vi "Measurement UI.vi"() -> ()   [LabVIEW 2022 SP3, in "Single Tone - Digital Mic UI.lvlib"]
uses:
  Single Tone - Digital Mic UI.lvlib
  shared/measurements/controls/measurement units.ctl
  shared/ui/controls/view.ctl
  shared/controls/input type.ctl
  UI State.ctl
  <vilib>/Utility/miscctls.llb/LVBoundsTypeDef.ctl
  <vilib>/Utility/miscctls.llb/LVPoint32TypeDef.ctl
  <vilib>/Utility/miscctls.llb/LVPointTypeDef.ctl
  shared/ui/UI Helpers.lvlib
  shared/configuration dialogs/Config Dialog.lvlib
panel:
  in  "view legend":T1
  out "time domain":waveform(dbl)[](graph)
  out "frequency domain":cluster{"x0":dbl, "dx":dbl, "magnitude":dbl[]}[](graph)
  out "meas table":string[][](table)
  out "THD":dbl caption="frequency (Hz) 3"
  out "THD+N":dbl caption="frequency (Hz) 2"
  out "SNR":dbl
  out "microphone sensitivity (dBFS)":dbl
  out "amplitude (dBSPL)":dbl
  out "amplitude (Pa RMS)":dbl
  out "frequency (Hz)":dbl
  out "channel name":string
  out "ref mic wfm - data":dbl[](array[numeric])
  out "ref mic wfm - dt":dbl
  in  "output channel":string="PXI1Slot4/ai0"
  in  "input cfg file":string
  in  "Configuration tab":enum32{"Input", "Measurement", "Units"}(tab)=enum."Measurement"
  in  "digital mic sensitivity (dBFS)":dbl=-26.0 caption="Microphone Sensitivity" format="%#.6p dBFS"
  out "input cfg file name":string
  in  "configure input":bool
  in  "digital channel list":string="PXI1Slot2\\PCMi 0" caption="Digital Audio Channel"
  in  "input type":T2 caption="Input Type"
  in  "Output Channel":tag="PXI1Slot2/ao0" caption="Channel"
  in  "output level (dBSPL)":dbl=94.0 caption="Output level" format="%#_3f dBSPL"
  in  "min settling cycles":u32 caption="Minimum settling cycles"
  in  "min settling time (s)":dbl=0.1 caption="Minimum settling time" format="%#_6ps"
  in  "min measurement cycles":u32 caption="Minimum measurement cycles"
  in  "min measurement time (s)":dbl=0.1 caption="Minimum measurement time" format="%#_6ps"
  in  "Ref Mic Channel":tag="PXI1Slot2/ai0" caption="Channel"
  in  "acq sampling rate":dbl=50.0 caption="Sensitivity" format="%#.6f mV/Pa"
  in  "lowpass filter":T3(ring) caption="Lowpass filter"
  in  "highpass filter":enum32{"DC", "AC"}(ring)=enum."AC" caption="Highpass filter"
  in  "band start":dbl=20.0 caption="Band start" format="%#_6pHz"
  in  "band stop":dbl=20000.0 caption="Band stop" format="%#_6pHz"
  in  "weighting filter":T4(ring)=enum."A-weighting" caption="Weighting filter"
  in  "output voltage ratio":dbl=3.39 caption="Output voltage ratio" format="%.3p Pa/V"
  in  "signal frequency":dbl=1000.0 caption="Frequency" format="%#_6pHz"
  in  "THD units":T5 caption="THD"
  in  "THD+N units":T5 caption="THD+N"
  in  "SNR units":T5 caption="SNR"
  out "fft - data":dbl[](array[numeric])
  out "fft - df":dbl
  out "fft - f0":dbl
  out "wfm - data":dbl[](array[numeric])
  out "wfm - dt":dbl
  in  "ref mic channel":string="PXI1Slot4/ai0"
  # "hidden controls - used to sync with MeasLink"
  # "hidden indicators"
  # "Digital Microphone Interface"
  # "Harware Resource"
  # "Output"
  # "Reference Microphone"
  # "Measurement Duration"
  # "Filters"
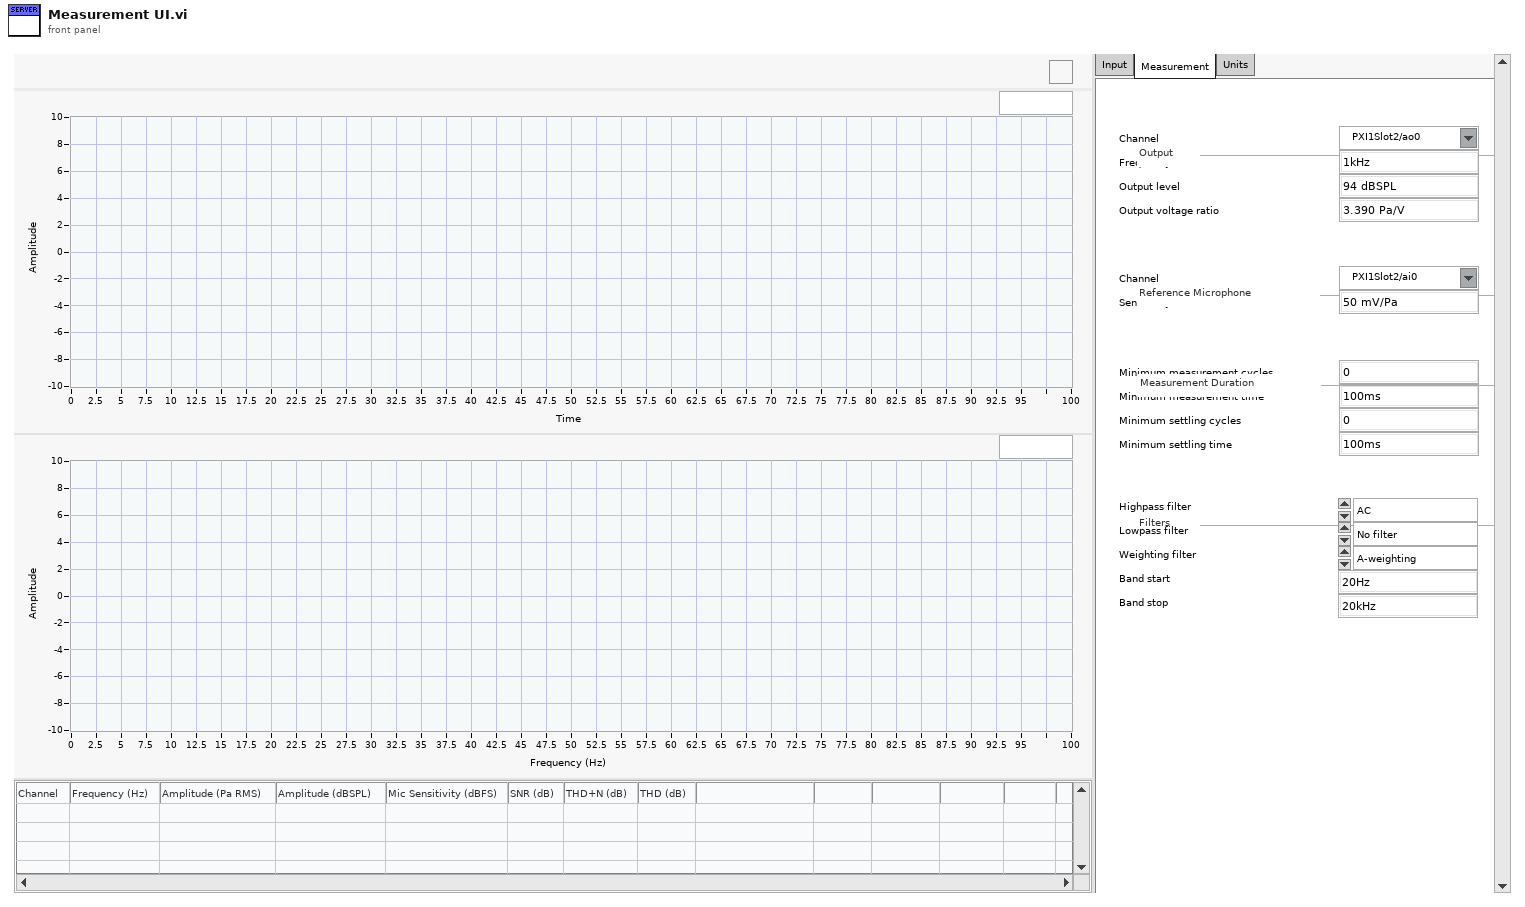
[diagram p1: front panel]
types:
  T1 = typedef "UI Helpers.lvlib/view.ctl" = bool
  T2 = typedef "input type.ctl" = enum32{"Digital Serial", "PDM"}
  T3 = enum32{"No filter", "AES17 20kHz", "AES17 40kHz"}
  T4 = enum32{"Linear", "A-weighting", "B-weighting", "C-weighting"}
  T5 = typedef "measurement units.ctl" = enum32{"dB", "%", "x/y"}
  T6 = typedef "Single Tone - Digital Mic UI.lvlib/UI State.ctl" = cluster{"Graph Size":T7, "Legend Visible":bool, "Mouse Coords":T8, "PostUI event occurred":bool, "input cfg file":path}
  T7 = typedef "LVBoundsTypeDef.ctl" = cluster{"Width":u32, "Height":u32}
  T8 = typedef "LVPoint32TypeDef.ctl" = cluster{"Horizontal":i32, "Vertical":i32}
  T9 = typedef "LVPointTypeDef.ctl" = cluster{"Horizontal":i16, "Vertical":i16}
  T10 = typedef "Config Dialog.lvlib/audio settings.ctl" = cluster{"input cfg file":string}
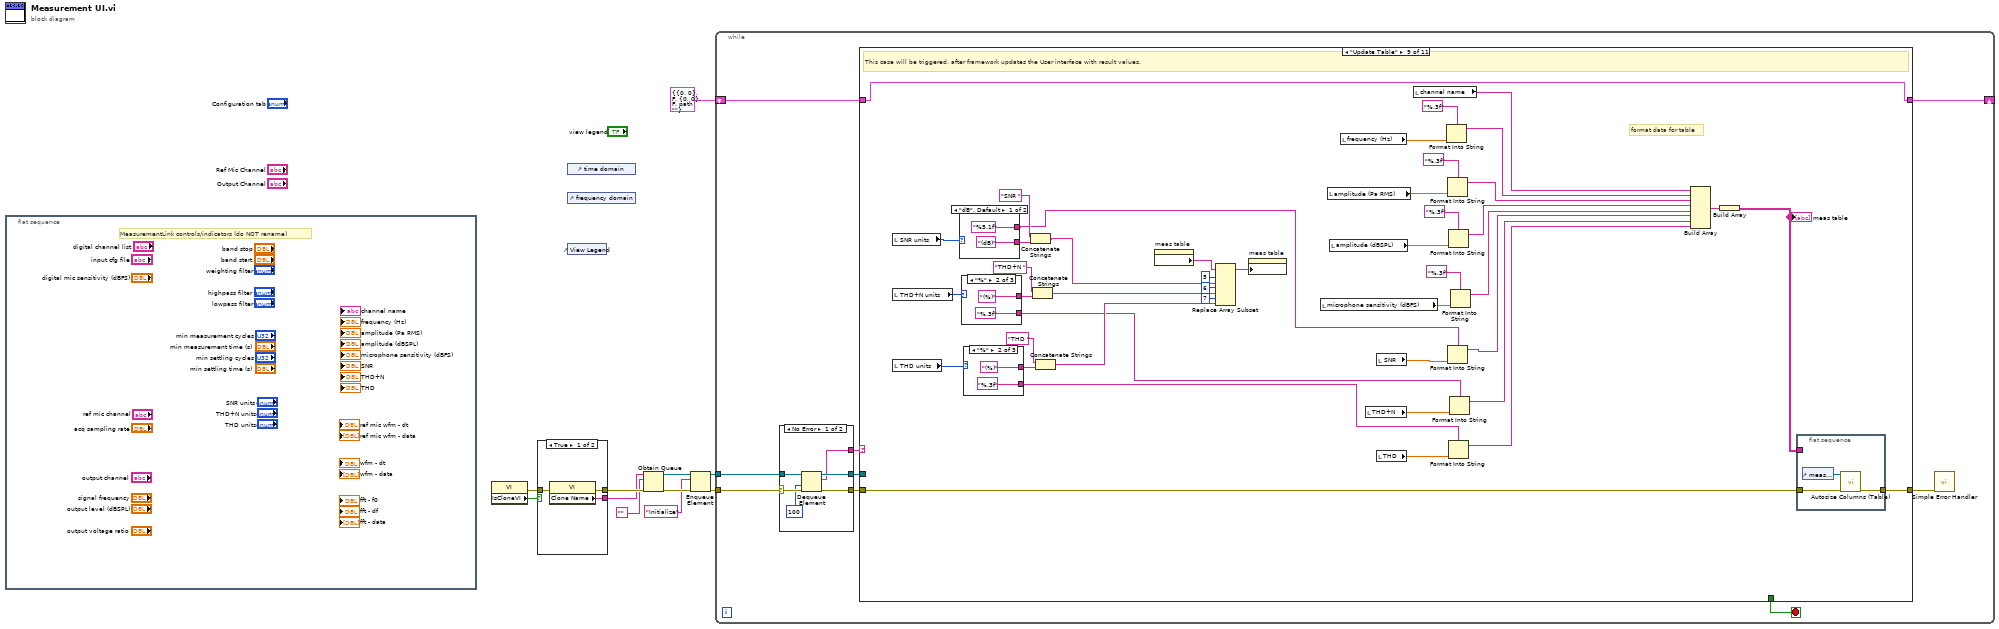
[diagram p0: block diagram]
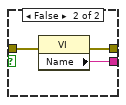
[diagram p2: hidden frame]
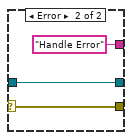
[diagram p3: hidden frame]
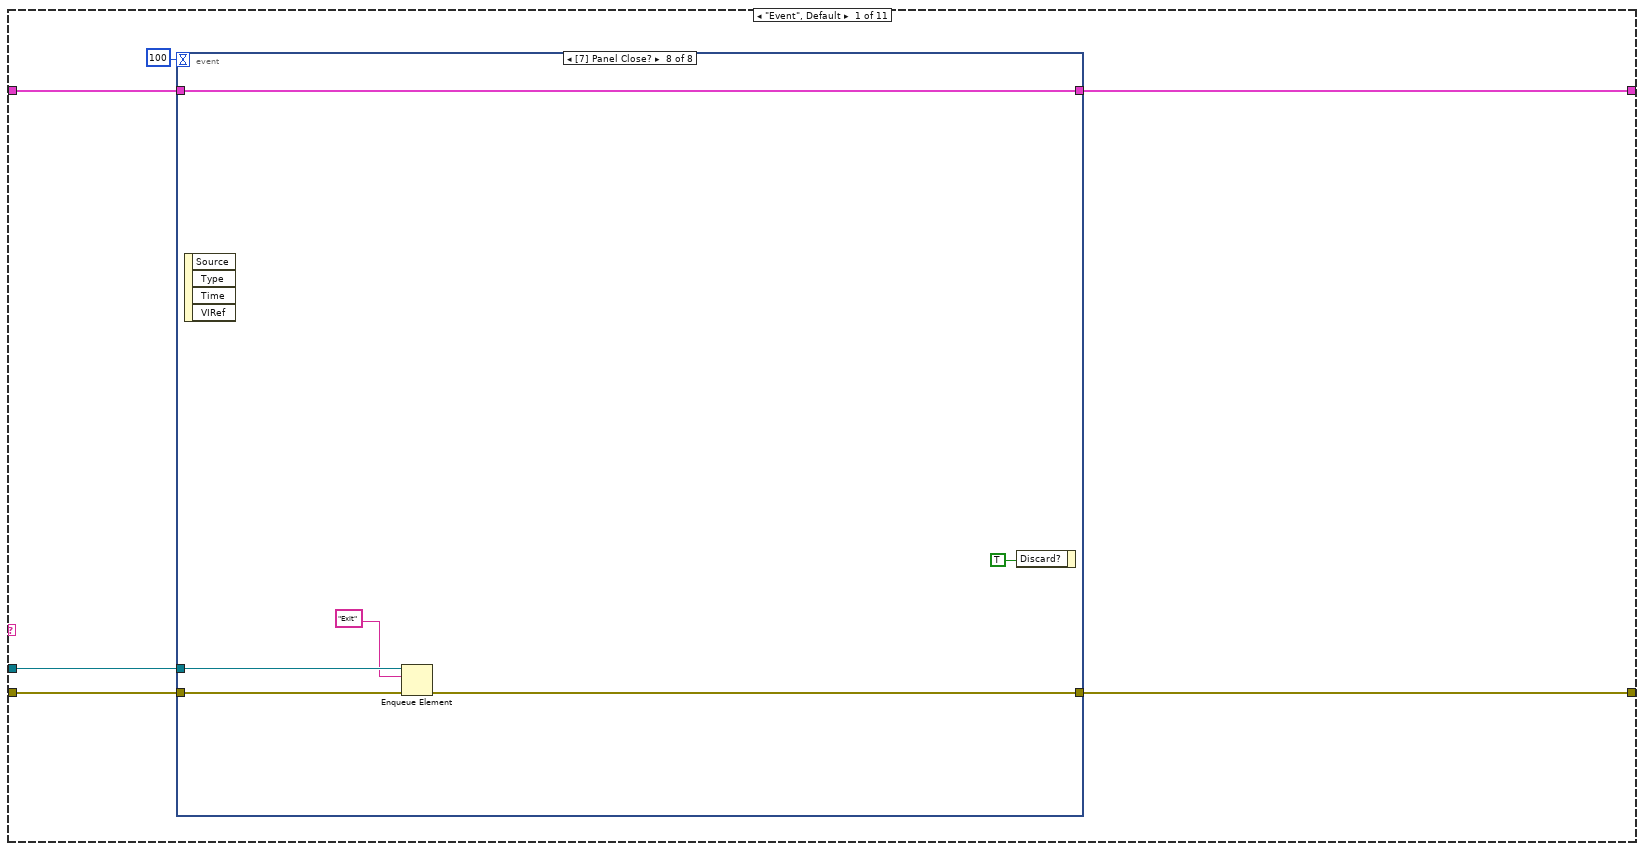
[diagram p4: hidden frame]
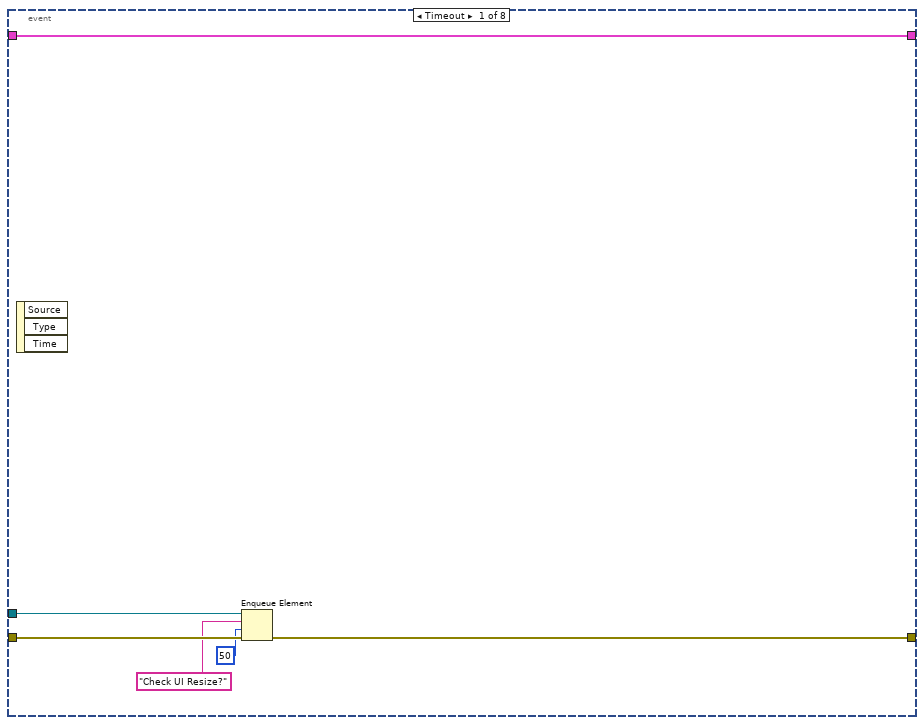
[diagram p5: hidden frame]
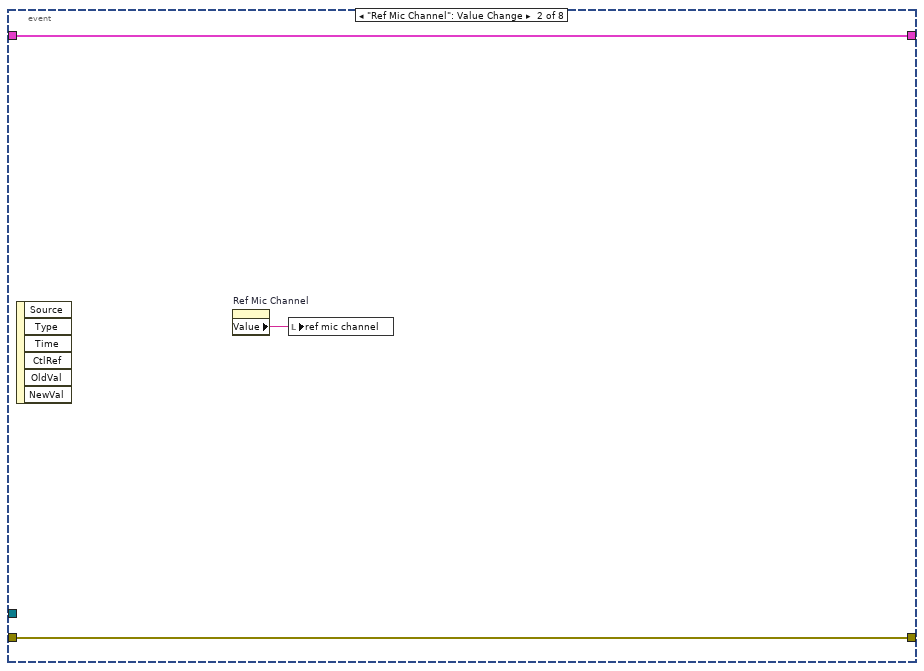
[diagram p6: hidden frame]
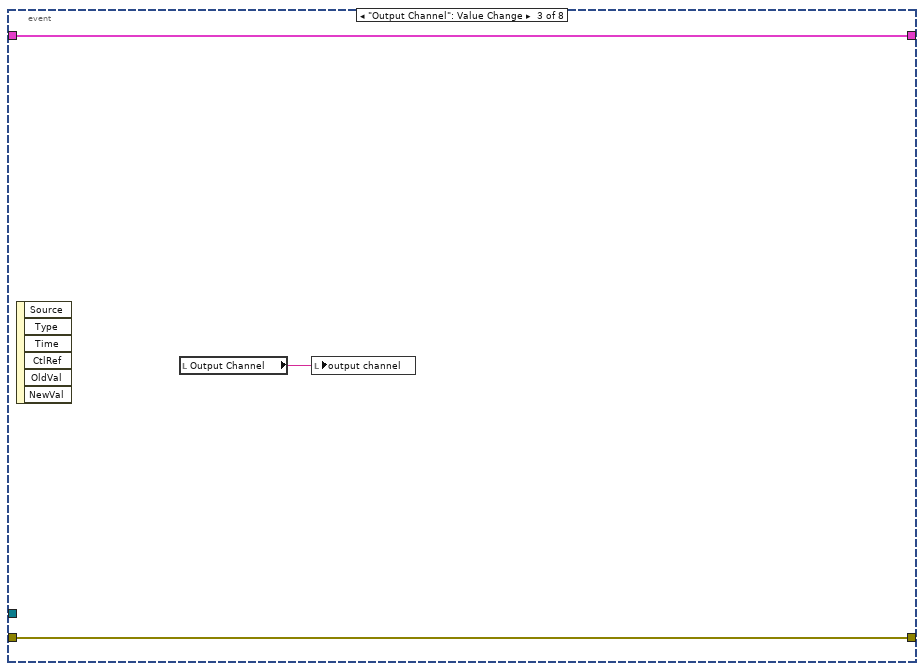
[diagram p7: hidden frame]
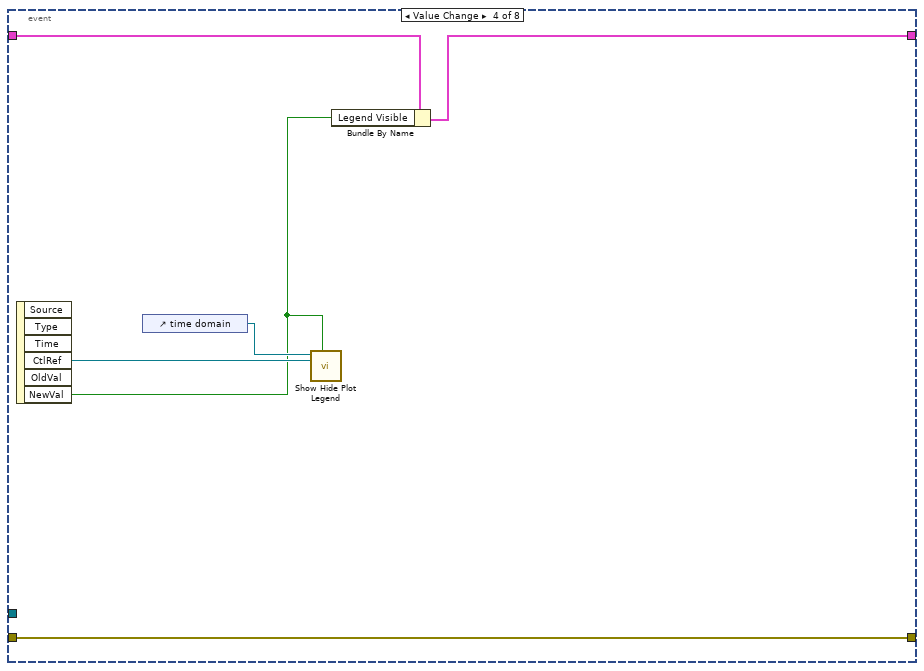
[diagram p8: hidden frame]
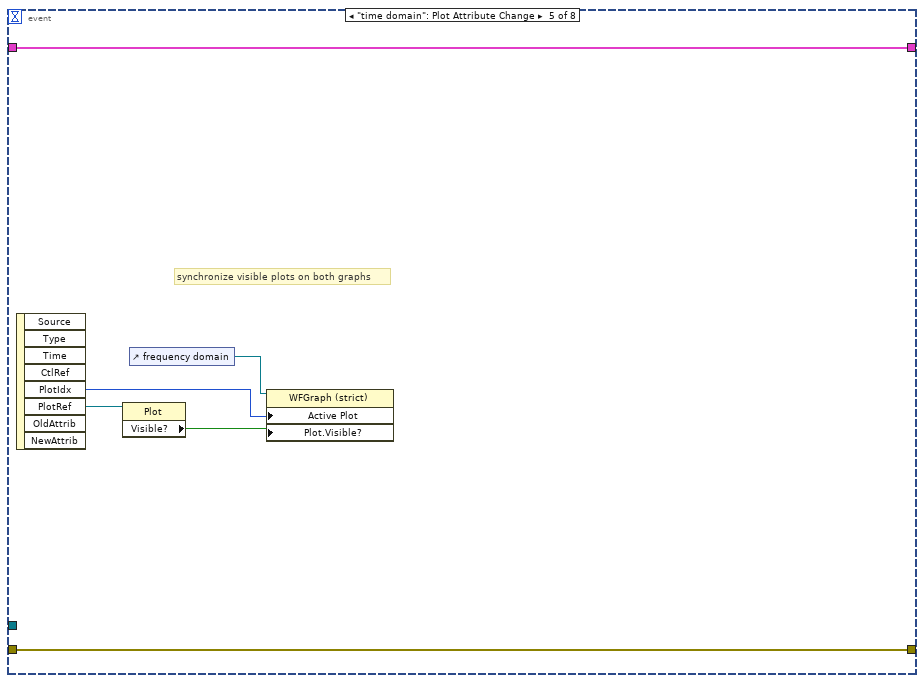
[diagram p9: hidden frame]
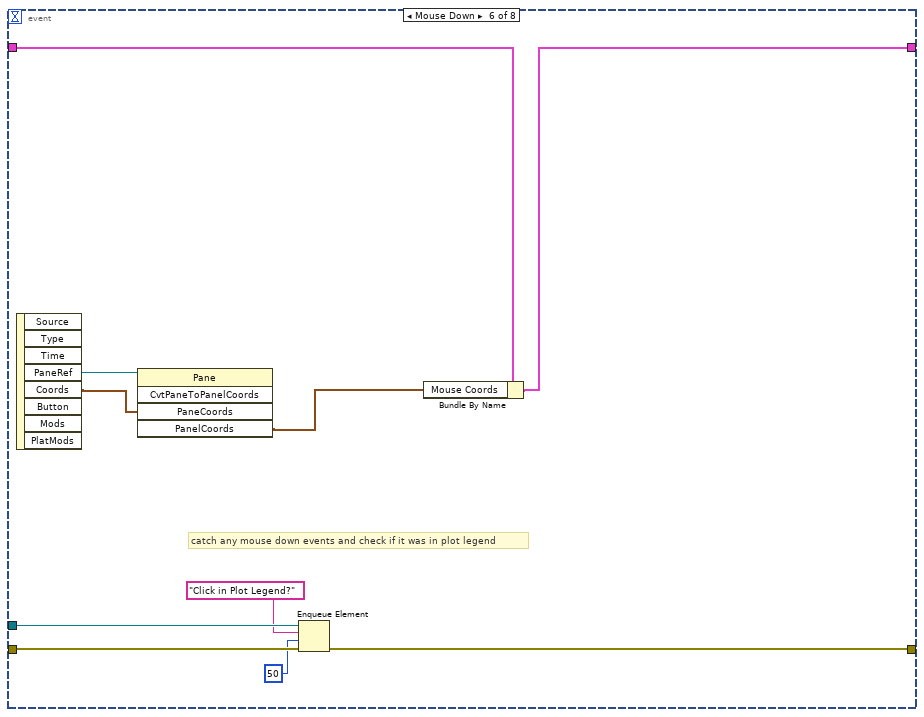
[diagram p10: hidden frame]
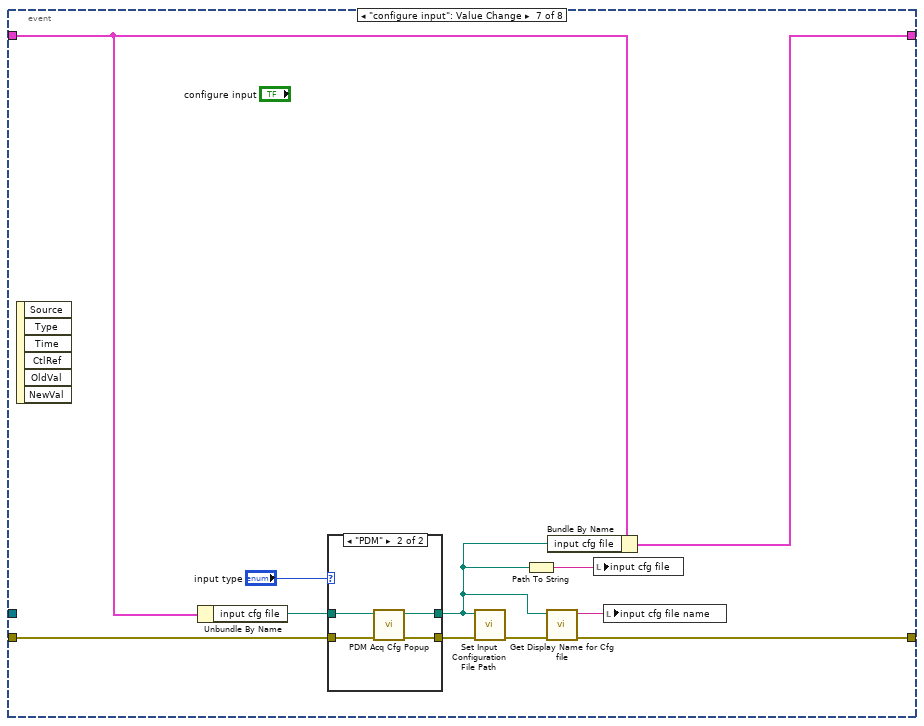
[diagram p11: hidden frame]
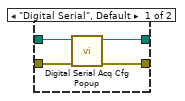
[diagram p12: hidden frame]
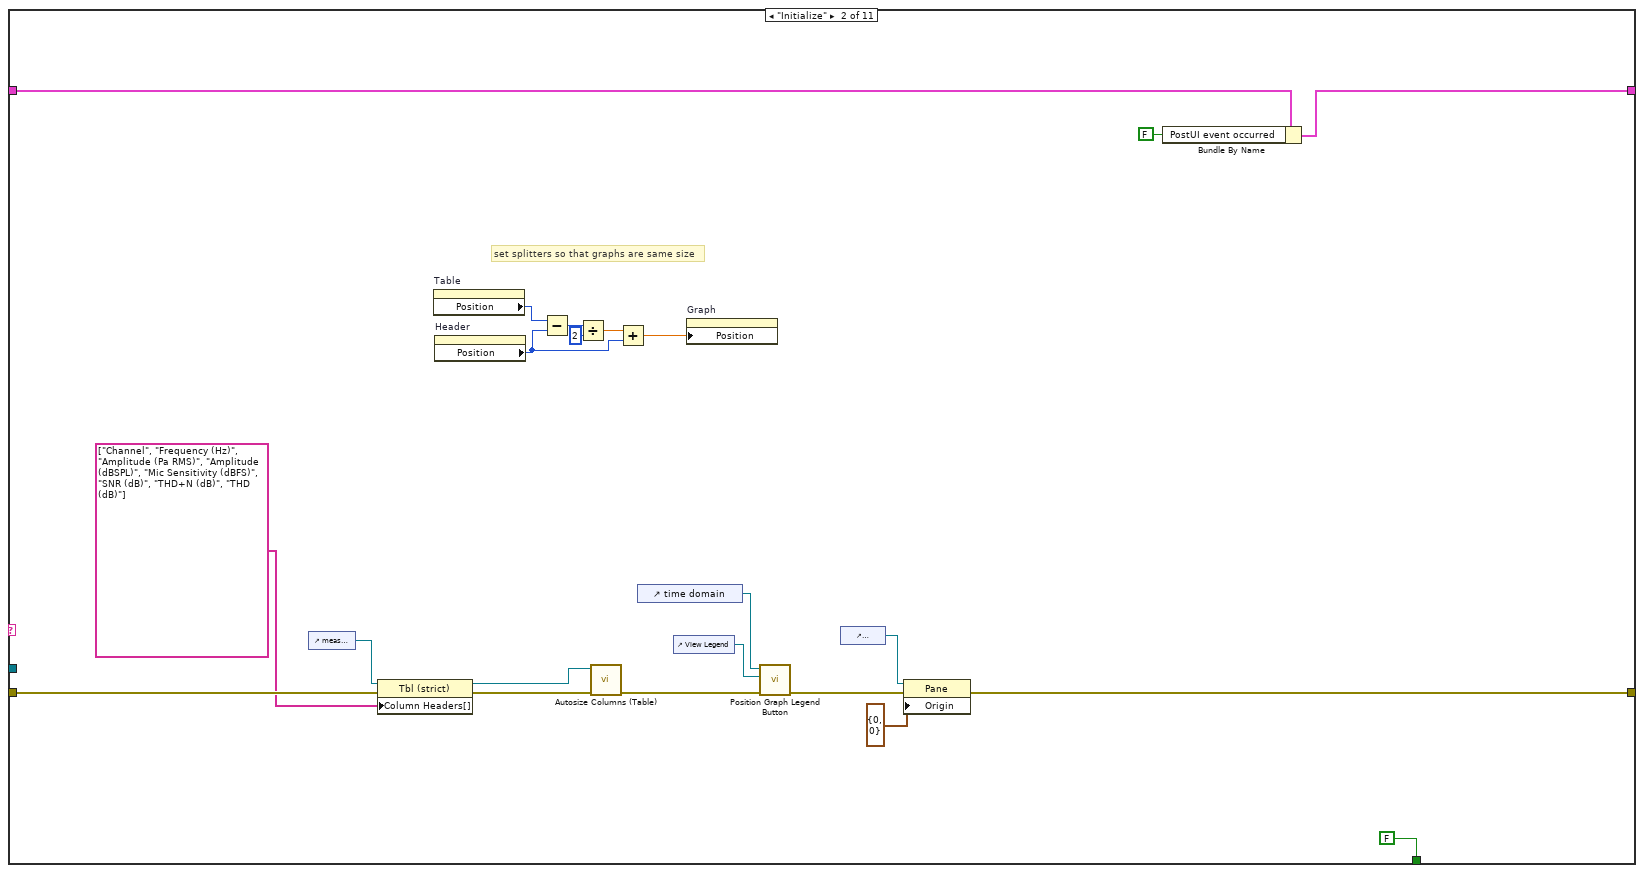
[diagram p13: hidden frame]
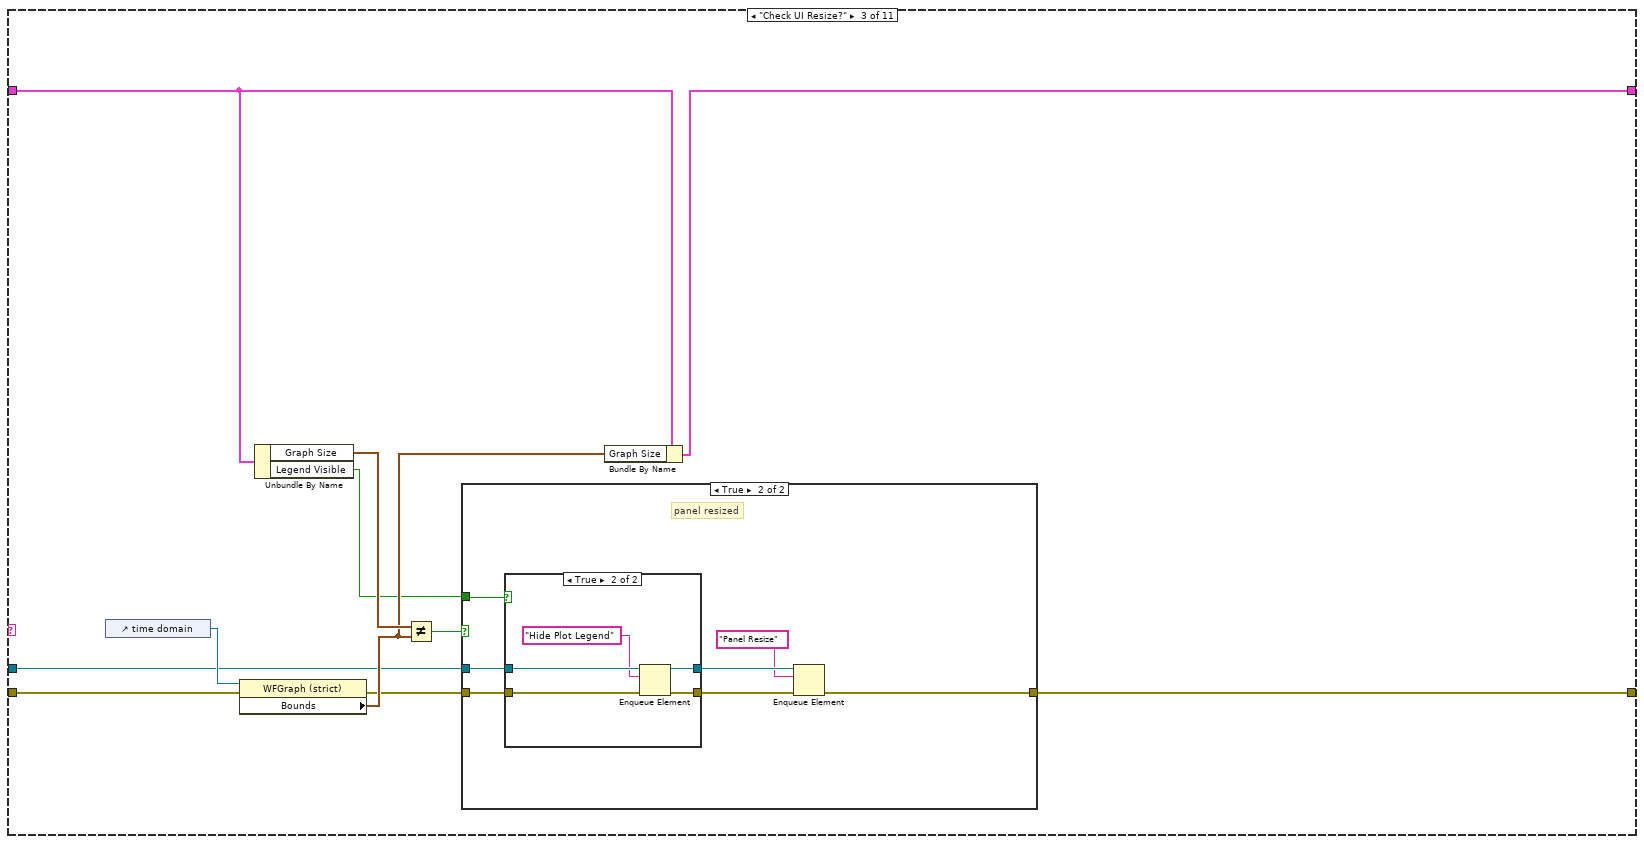
[diagram p14: hidden frame]
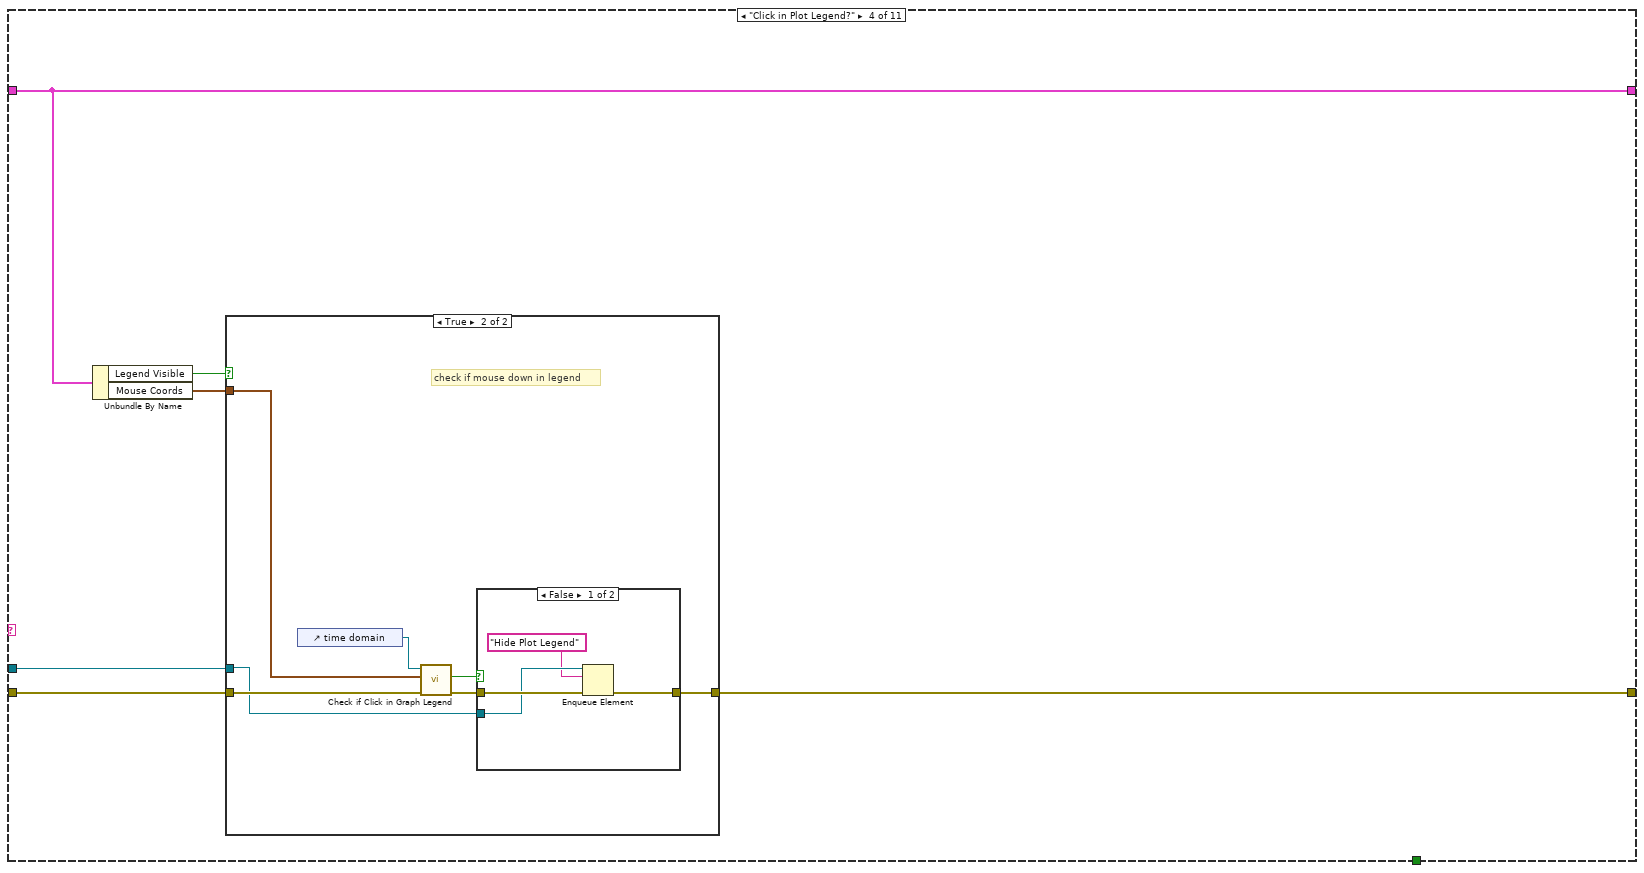
[diagram p17: hidden frame]
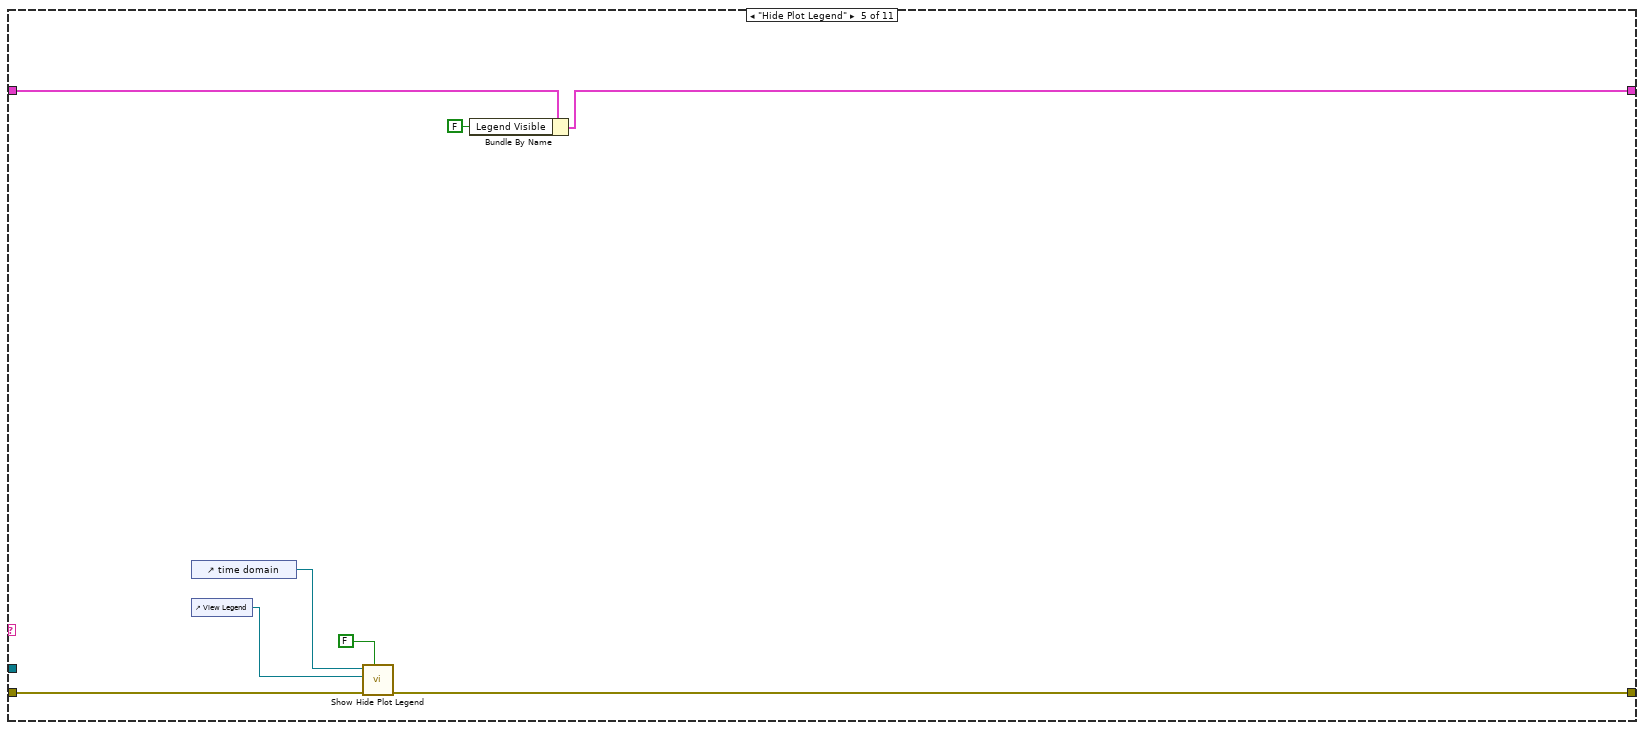
[diagram p20: hidden frame]
diagram:
  n1 = flat-sequence {
    frame #0 {
      # "MeasurementLink controls/indicators (do NOT rename)"
    }
  }
  n2 = property class="VI"() -> (error out=w2:errorcluster, "IsCloneVI"=w3:bool)  [unwired: 2 in, 1 out]
  n3 = case shown="True" w3 {
    tunnel: [w14 w17] -> w11
    tunnel: [w13 w16] -> w10
    tunnel: w2 -> [w12 w15]
    frame True {
      n4 = property class="VI"(error in=w12) -> (error out=w14:errorcluster, "Clone Name"=w13:string)  [unwired: 1 in, 1 out]
    }
    frame False {
      n5 = property class="VI"(error in=w15) -> (error out=w17:errorcluster, "Name"=w16:string)  [unwired: 1 in, 1 out]
    }
  }
  n6 = control-ref of="time domain"() -> ()  [unwired: 1 out]
  n7 = control-ref of="frequency domain"() -> ()  [unwired: 1 out]
  n8 = control-ref of="View Legend"() -> ()  [unwired: 1 out]
  n9 = Obtain Queue(name (unnamed)=w10, element data type="", error in (no error)=w11) -> (queue out=w7:refnum<queue>, error out=w9:errorcluster)  [unwired: 2 in, 1 out]
  n10 = Enqueue Element(queue=w7, element="Initialize", error in (no error)=w9) -> (queue out=w6:refnum<queue>, error out=w8:errorcluster)  [unwired: 1 in, 1 out]
  n11 = while {
    tunnel: w6 -> [w24]
    shift-right: [w20] -> _
    shift-left: T6 {"Graph Size"={"Width"=0, "Height"=0}, "Legend Visible"=FALSE, "Mouse Coords"={"Horizontal"=0, "Vertical"=0}, "PostUI event occurred"=FALSE, "input cfg file"=path ""} ("ui state") -> [w19]
    tunnel: w8 -> [w26]
    stop <- w21 stop-if-true
    n12 = case shown="No Error" w26 {
      selector: w26 -> [w32 w35]
      tunnel: [w31 w35] -> w25
      tunnel: w24 -> [w30 w34]
      tunnel: [w29 w34] -> w23
      tunnel: [w28 "Handle Error"] -> w22
      frame No Error {
        n13 = Dequeue Element(queue=w30, timeout in ms (-1)=100, error in (no error)=w32) -> (queue out=w29:refnum<queue>, element=w28:string, error out=w31:errorcluster)  [unwired: 1 out]
      }
      frame Error {
      }
    }
    n14 = case shown="\"Update Table\"" w22 {
      tunnel: w25 -> [w40 w118 w132 w150 w172 w177 w188 w228 w238 w306 w308]
      tunnel: w23 -> [w38 _ w123 w151 _ _ w187 _ _ w304 _]
      tunnel: [w41 w104 w125 w149 w171 w176 w183 w228 w241 w301 w308] -> w18
      tunnel: [_ FALSE _ _ _ _ _ _ _ TRUE _] -> w21
      tunnel: [w36 w102 w128 w154 w173 w180 w181 w229 w239 w299 w307] -> w20
      tunnel: w19 -> [w37 w103 w129 w154 w174 w180 w182 w229 w239 w299 w307]
      frame "Event", Default {
        n15 = event shown="[7] Panel Close?" {
          selector: _ -> [_ _ _ _ _ _ _ _]
          dyn-events: _ -> [_ _ _ _ _ _ _ _]
          timeout: 100 -> [_ _ _ _ _ _ _ _]
          tunnel: [w44 w48 w53 w56 w60 w73 w83 w98] -> w41
          tunnel: w40 -> [w47 w48 w53 w56 w60 w74 w81 w99]
          tunnel: w38 -> [w46 _ _ _ _ w75 _ w97]
          tunnel: w37 -> [w43 w49 w52 w58 w61 w70 w85 w95]
          tunnel: [w43 w49 w52 w57 w61 w69 w84 w95] -> w36
          event Timeout {
            n16 = event-data() -> ()  [unwired: 1 in, 3 out]
            n17 = Enqueue Element(queue=w46, element="Check UI Resize?", timeout in ms (-1)=50, error in (no error)=w47) -> (error out=w44:errorcluster)  [unwired: 2 out]
          }
          event "Ref Mic Channel": Value Change {
            n18 = event-data() -> ()  [unwired: 1 in, 6 out]
            n19 = property on="Ref Mic Channel" class="DAQmxName"() -> ("Value"=w50:string)  [unwired: 2 in, 2 out]
            n20 = local write "ref mic channel"(w50) -> ()
          }
          event "Output Channel": Value Change {
            n21 = event-data() -> ()  [unwired: 1 in, 6 out]
            n22 = local read "Output Channel"() -> (w51:tag)
            n23 = local write "output channel"(w51) -> ()
          }
          event Value Change {
            n24 = event-data() -> ("CtlRef"=w55:refnum<vi>, "NewVal"=w54:T1)  [unwired: 1 in, 4 out]
            n25 = control-ref of="time domain"() -> (w59:refnum<vi>)
            n26 = call "Show Hide Plot Legend.vi"("show"=w54, "view reference"=w55, "graph reference"=w59) -> ()  [unwired: 8 in, 1 out]
            n27 = Bundle By Name(cluster=w58, "Legend Visible"=w54) -> (w57:T6)
          }
          event "time domain": Plot Attribute Change {
            # "synchronize visible plots on both graphs"
            n28 = event-data() -> ("PlotIdx"=w63:i32, "PlotRef"=w64:refnum<vi>)  [unwired: 1 in, 6 out]
            n29 = property class="Plot"(reference=w64) -> ("Visible?"=w65:bool)  [unwired: 1 in, 2 out]
            n30 = control-ref of="frequency domain"() -> (w62:refnum<vi>)
            n31 = property on="Property Node" class="WFGraph (strict)"(reference=w62, "Active Plot"=w63, "Plot.Visible?"=w65) -> ()  [unwired: 1 in, 2 out]
          }
          event Mouse Down {
            # "catch any mouse down events and check if it was in plot legend"
            n32 = event-data() -> ("PaneRef"=w68:refnum<vi>, "Coords"=w67:T8)  [unwired: 1 in, 6 out]
            n33 = invoke class="Pane" method="CvtPaneToPanelCoords"(reference=w68, "PaneCoords"=w67) -> ("PanelCoords"=w66:T9)  [unwired: 3 in, 4 out]
            n34 = Enqueue Element(queue=w75, element="Click in Plot Legend?", timeout in ms (-1)=50, error in (no error)=w74) -> (error out=w73:errorcluster)  [unwired: 2 out]
            n35 = Bundle By Name(cluster=w70, "Mouse Coords"=w66) -> (w69:T6)
          }
          event "configure input": Value Change {
            n36 = event-data() -> ()  [unwired: 1 in, 6 out]
            n37 = Unbundle By Name(w85) -> ("input cfg file"=w82:path)
            n38 = case shown="\"PDM\"" "input type" {
              tunnel: w82 -> [w90 w94]
              tunnel: w81 -> [w89 w93]
              tunnel: [w88 w91] -> w80
              tunnel: [w87 w92] -> w78
              frame "Digital Serial", Default {
                n39 = call "Digital Serial Acq Cfg Popup.vi"("error in (no error)"=w89, "config file in"=w90) -> ("error out"=w88:errorcluster, "config file out"=w87:path)  [unwired: 7 in, 1 out]
              }
              frame "PDM" {
                n40 = call "PDM Acq Cfg Popup.vi"("error in (no error)"=w93, "config file in"=w94) -> ("error out"=w91:errorcluster, "config file out"=w92:path)  [unwired: 7 in, 1 out]
              }
            }
            n41 = call "Set Input Configuration File Path.vi"("error in (no error)"=w80, "configuration file"=w78) -> ("error out"=w79:errorcluster)  [unwired: 9 in]
            n42 = Path To String(path=w78) -> (string=w86:string)
            n43 = call "Get Display Name for Cfg file.vi"("error in (no error)"=w79, "file path"=w78) -> ("error out"=w83:errorcluster, "display string"=w77:string)  [unwired: 8 in]
            n44 = Bundle By Name(cluster=w85, "input cfg file"=w78) -> (w84:T6)
            n45 = local write "input cfg file"(w86) -> ()
            n46 = local write "input cfg file name"(w77) -> ()
          }
          event Panel Close? {
            n47 = event-data() -> ()  [unwired: 1 in, 4 out]
            n48 = Enqueue Element(queue=w97, element="Exit", error in (no error)=w99) -> (error out=w98:errorcluster)  [unwired: 1 in, 2 out]
            n49 = event-data("Discard?"=TRUE) -> ()  [unwired: 1 in, 1 out]
          }
        }
      }
      frame "Initialize" {
        # "set splitters so that graphs are same size"
        n50 = control-ref of="meas table"() -> (w116:refnum<vi>)
        n51 = property class="Tbl (strict)"(reference=w116, error in=w118, "Column Headers[]"=string[] ["Channel", "Frequency (Hz)", "Amplitude (Pa RMS)", "Amplitude (dBSPL)", "Mic Sensitivity (dBFS)", "SNR (dB)", "THD+N (dB)", "THD (dB)"] ("Column Header Strings[]")) -> (reference out=w115:refnum<vi>, error out=w117:errorcluster)
        n52 = property on="Table" class="Splitter"() -> ("Position"=w113:i32)  [unwired: 2 in, 2 out]
        n53 = property on="Header" class="Splitter"() -> ("Position"=w109:i32)  [unwired: 2 in, 2 out]
        n54 = Subtract(x=w113, y=w109) -> (x-y=w112:i32)
        n55 = Divide(x=w112, y=2) -> (x/y=w110:dbl)
        n56 = call "Autosize Columns (Table).vi"("error in (no error)"=w117, "table"=w115) -> ("error out"=w119:errorcluster)  [unwired: 9 in]
        n57 = Add(x=w110, y=w109) -> (x+y=w108:dbl)
        n58 = control-ref of="time domain"() -> (w121:refnum<vi>)
        n59 = control-ref of="View Legend"() -> (w120:refnum<vi>)
        n60 = property on="Graph" class="Splitter"("Position"=w108) -> ()  [unwired: 2 in, 2 out]
        n61 = call "Position Graph Legend Button.vi"("error in (no error)"=w119, "view legend"=w120, "graph"=w121) -> ("error out"=w107:errorcluster)  [unwired: 8 in]
        n62 = control-ref of="Configuration"() -> (w106:refnum<vi>)
        n63 = property class="Pane"(reference=w106, error in=w107, "Origin"=T9 {"Horizontal"=0, "Vertical"=0}) -> (error out=w104:errorcluster)  [unwired: 1 out]
        n64 = Bundle By Name(cluster=w103, "PostUI event occurred"=FALSE) -> (w102:T6)
      }
      frame "Check UI Resize?" {
        n65 = control-ref of="time domain"() -> (w133:refnum<vi>)
        n66 = property on="Property Node" class="WFGraph (strict)"(reference=w133, error in=w132) -> (error out=w126:errorcluster, "Bounds"=w130:T7)  [unwired: 1 out]
        n67 = Unbundle By Name(w129) -> ("Graph Size"=w131:T7, "Legend Visible"=w124:bool)
        n68 = Not Equal?(x=w131, y=w130) -> (x != y?=w127:bool)
        n69 = case shown="True" w127 {
          tunnel: w126 -> [w134 w141]
          tunnel: [w134 w136] -> w125
          tunnel: w124 -> [_ w139]
          tunnel: w123 -> [_ w140]
          frame False {
            # "no resize"
          }
          frame True {
            # "panel resized"
            n70 = case shown="True" w139 {
              tunnel: w141 -> [w143 w148]
              tunnel: [w143 w147] -> w138
              tunnel: w140 -> [w142 w146]
              tunnel: [w142 w144] -> w137
              frame False {
              }
              frame True {
                n71 = Enqueue Element(queue=w146, element="Hide Plot Legend", error in (no error)=w148) -> (queue out=w144:refnum<queue>, error out=w147:errorcluster)  [unwired: 1 in, 1 out]
              }
            }
            n72 = Enqueue Element(queue=w137, element="Panel Resize", error in (no error)=w138) -> (error out=w136:errorcluster)  [unwired: 1 in, 2 out]
          }
        }
        n73 = Bundle By Name(cluster=w129, "Graph Size"=w130) -> (w128:T6)
      }
      frame "Click in Plot Legend?" {
        n74 = Unbundle By Name(w154) -> ("Legend Visible"=w153:bool, "Mouse Coords"=w152:T8)
        n75 = case shown="True" w153 {
          tunnel: w152 -> [_ w160]
          tunnel: w151 -> [_ w157]
          tunnel: w150 -> [w155 w162]
          tunnel: [w155 w156] -> w149
          frame False {
            # "legend not visible; do nothing"
          }
          frame True {
            # "check if mouse down in legend"
            n76 = control-ref of="time domain"() -> (w161:refnum<vi>)
            n77 = call "Check if Click in Graph Legend.vi"("error in (no error)"=w162, "Mouse Coords"=w160, "WaveformGraph"=w161) -> ("error out"=w158:errorcluster, "click in legend?"=w159:bool)  [unwired: 7 in]
            n78 = case shown="False" w159 {
              tunnel: w158 -> [w166 w167]
              tunnel: w157 -> [w165 _]
              tunnel: [w164 w167] -> w156
              frame False {
                n79 = Enqueue Element(queue=w165, element="Hide Plot Legend", error in (no error)=w166) -> (error out=w164:errorcluster)  [unwired: 1 in, 2 out]
              }
              frame True {
                # "inside legend; do nothing"
              }
            }
          }
        }
      }
      frame "Hide Plot Legend" {
        n80 = control-ref of="time domain"() -> (w169:refnum<vi>)
        n81 = control-ref of="View Legend"() -> (w168:refnum<vi>)
        n82 = call "Show Hide Plot Legend.vi"("show"=FALSE, "error in (no error)"=w172, "view reference"=w168, "graph reference"=w169) -> ("error out"=w171:errorcluster)  [unwired: 7 in]
        n83 = Bundle By Name(cluster=w174, "Legend Visible"=FALSE ("legend visible")) -> (w173:T6)
      }
      frame "Panel Resize" {
        n84 = control-ref of="time domain"() -> (w179:refnum<vi>)
        n85 = control-ref of="View Legend"() -> (w178:refnum<vi>)
        n86 = call "Position Graph Legend Button.vi"("error in (no error)"=w177, "view legend"=w178, "graph"=w179) -> ("error out"=w176:errorcluster)  [unwired: 8 in]
      }
      frame "Post UI Update" {
        # "This case will be triggered, after framework updates the User interface with result values."
        n87 = for {
          tunnel: w187 -> [w212]
          shift-right: [w211] -> w184
          shift-left: w188 -> [w213]
          tunnel: string[] ["Update Table", "Update Graphs"] -> [w210] mode=indexing
          n88 = Enqueue Element(queue=w212, element=w210, timeout in ms (-1)=50, error in (no error)=w213) -> (error out=w211:errorcluster)  [unwired: 2 out]
        }
        n89 = Unbundle By Name(w182) -> ("PostUI event occurred"=w185:bool)
        n90 = case shown="False" w185 {
          tunnel: w184 -> [w196 w209]
          tunnel: [w191 w209] -> w183
          tunnel: w182 -> [w199 w208]
          tunnel: [w198 w208] -> w181
          frame False {
            # "do this on first PostUI Event (happens when panel loads)"
            # "Initialize the DAQmx channel control"
            n91 = local read "ref mic channel"() -> (w201:string)
            n92 = local read "output channel"() -> (w189:string)
            n93 = local read "input cfg file"() -> (w195:string)
            n94 = property on="Ref Mic Channel" class="DAQmxName"("Value"=w201) -> ()  [unwired: 2 in, 2 out]
            n95 = property on="Output Channel" class="DAQmxName"("Value"=w189) -> ()  [unwired: 2 in, 2 out]
            n96 = Empty String/Path?(string/path=w195) -> (empty?=w197:bool)
            n97 = case shown="True" w197 {
              tunnel: w196 -> [w203 w207]
              tunnel: [w203 w205] -> w194
              tunnel: w195 -> [w202 _]
              tunnel: [w202 w204] -> w190
              frame False {
              }
              frame True {
                n98 = call "Get Audio Settings.vi"("error in (no error)"=w207) -> ("error out"=w205:errorcluster, "audio settings"=w206:T10)  [unwired: 9 in]
                n99 = Unbundle By Name(w206) -> ("input cfg file"=w204:string)
              }
            }
            n100 = String To Path(string=w190) -> (path=w193:path)
            n101 = call "Get Display Name for Cfg file.vi"("error in (no error)"=w194, "file path"=w193) -> ("error out"=w191:errorcluster, "display string"=→"input cfg file name":string)  [unwired: 8 in]
            n102 = Bundle By Name(cluster=w199, "PostUI event occurred"=TRUE, "input cfg file"=w193) -> (w198:T6)
            n103 = local write "input cfg file"(w190) -> ()
          }
          frame True {
          }
        }
      }
      frame "Update Graphs" {
        # "This case will be triggered, after framework updates the User interface with result values."
        n104 = local read "channel name"() -> (w216:string)
        n105 = control-ref of="time domain"() -> (w227:refnum<vi>)
        n106 = control-ref of="frequency domain"() -> (w224:refnum<vi>)
        n107 = local read "wfm - data"() -> (w222:dbl[])
        n108 = local read "wfm - dt"() -> (w221:dbl)
        n109 = local read "fft - data"() -> (w219:dbl[])
        n110 = local read "fft - df"() -> (w217:dbl)
        n111 = local read "fft - f0"() -> (w218:dbl)
        n112 = Build Array(w216) -> (w215:string[])
        n113 = call "Array to Wfm (N Ch).vi"("channel names"=w215, "dt"=w221, "array"=w222) -> ("waveforms"=→"time domain":waveform(dbl)[])  [unwired: 8 in]
        n114 = call "Array to Spectra (N Ch).vi"("channel names"=w215, "df"=w217, "f0"=w218, "data"=w219) -> ("spectra"=→"frequency domain":cluster{"f0":dbl, "df":dbl, "data":dbl[]}[])  [unwired: 7 in]
        n115 = for {
          tunnel: w224 -> [w230]
          tunnel: w215 -> [_] mode=indexing
          i -> [w231]
          # "make all plots visible"
          n116 = property class="WFGraph (strict)"(reference=w230, "Active Plot"=w231, "Plot.Visible?"=TRUE ("Plot.Visible")) -> ()  [unwired: 1 in, 2 out]
        }
        n117 = for {
          tunnel: w227 -> [w233]
          tunnel: w215 -> [_] mode=indexing
          i -> [w234]
          # "make all plots visible"
          n118 = property class="WFGraph (strict)"(reference=w233, "Active Plot"=w234, "Plot.Visible?"=TRUE ("Plot.Visible")) -> ()  [unwired: 1 in, 2 out]
        }
        n119 = Array Size(array=w215) -> (size(s)=w226:i32)
        n120 = property class="WFGraph (strict)"(reference=w227, "LegNumRows"=w226, "LegScrollVis"=FALSE ("Legend:Scrollbar Visible")) -> ()  [unwired: 1 in, 2 out]
      }
      frame "Update Table" {
        # "format data for table"
        # "This case will be triggered, after framework updates the User interface with result values."
        n121 = local read "SNR units"() -> (w266:T5)
        n122 = local read "THD+N units"() -> (w276:T5)
        n123 = local read "THD units"() -> (w264:T5)
        n124 = case shown="\"dB\", Default" w266 {
          tunnel: ["(dB)" "(ratio)"] -> w275
          tunnel: ["%5.1f" ("initial string") "%.1f" ("initial string")] -> w262
          frame "dB", Default {
          }
          frame "x/y" {
          }
        }
        n125 = case shown="\"%\"" w276 {
          tunnel: ["(dB)" "(%)" "(ratio)"] -> w278
          tunnel: ["%5.1f" ("initial string") "%.3f" ("initial string") "%.6f" ("initial string")] -> w259
          frame "dB", Default {
          }
          frame "%" {
          }
          frame "x/y" {
          }
        }
        n126 = case shown="\"%\"" w264 {
          tunnel: ["(dB)" "(%)" "(ratio)"] -> w265
          tunnel: ["%5.1f" ("initial string") "%.3f" ("initial string") "%.6f" ("initial string")] -> w256
          frame "dB", Default {
          }
          frame "%" {
          }
          frame "x/y" {
          }
        }
        n127 = Concatenate Strings("SNR " ("string"), w275) -> (w272:string)
        n128 = Concatenate Strings("THD+N " ("string"), w278) -> (w271:string)
        n129 = Concatenate Strings("THD " ("string"), w265) -> (w270:string)
        n130 = property on="meas table" class="Tbl (strict)"() -> ("Column Headers[]"=w242:string[])  [unwired: 2 in, 2 out]
        n131 = Replace Array Subset(array=w242, new element #1=w272, index #1=5 ("index"), new element #2=w271, index #2=6 ("index"), new element #3=w270, index #3=7 ("index")) -> (w273:string[])
        n132 = property on="meas table" class="Tbl (strict)"("Column Headers[]"=w273) -> ()  [unwired: 2 in, 2 out]
        n133 = local read "microphone sensitivity (dBFS)"() -> (w243:dbl)
        n134 = local read "amplitude (Pa RMS)"() -> (w250:dbl)
        n135 = local read "amplitude (dBSPL)"() -> (w247:dbl)
        n136 = local read "frequency (Hz)"() -> (w253:dbl)
        n137 = local read "THD+N"() -> (w261:dbl)
        n138 = local read "THD"() -> (w258:dbl)
        n139 = local read "SNR"() -> (w263:dbl)
        n140 = local read "channel name"() -> (w240:string)
        n141 = Format Into String(format string="%.3f" ("initial string"), w253) -> (resulting string=w252:string)  [unwired: 2 in, 1 out]
        n142 = Format Into String(format string="%.3f" ("initial string"), w250) -> (resulting string=w249:string)  [unwired: 2 in, 1 out]
        n143 = Format Into String(format string=w262, w263) -> (resulting string=w255:string)  [unwired: 2 in, 1 out]
        n144 = Format Into String(format string="%.3f" ("initial string"), w247) -> (resulting string=w246:string)  [unwired: 2 in, 1 out]
        n145 = Format Into String(format string=w256, w258) -> (resulting string=w257:string)  [unwired: 2 in, 1 out]
        n146 = Format Into String(format string=w259, w261) -> (resulting string=w260:string)  [unwired: 2 in, 1 out]
        n147 = Format Into String(format string="%.3f" ("initial string"), w243) -> (resulting string=w244:string)  [unwired: 2 in, 1 out]
        n148 = Build Array(w240, w252, w249, w246, w244, w255, w260, w257) -> (w237:string[])
        n149 = Build Array(w237) -> (w236:string[][])
        "meas table" <- w236
        n150 = flat-sequence {
          tunnel: [w282] -> w241
          tunnel: w236 -> [_]
          tunnel: w238 -> [w280]
          frame #0 {
            n151 = control-ref of="meas table"() -> (w281:refnum<vi>)
            n152 = call "Autosize Columns (Table).vi"("error in (no error)"=w280, "table"=w281) -> ("error out"=w282:errorcluster)  [unwired: 9 in]
          }
        }
      }
      frame "Exit" {
        # "This case is triggered to close the User Interface from framework"
        n153 = Flush Queue(queue=w304, error in (no error)=w306) -> (queue out=w303:refnum<queue>, error out=w302:errorcluster)  [unwired: 1 out]
        n154 = Release Queue(queue=w303, force destroy? (F)=TRUE, error in (no error)=w302) -> (error out=w301:errorcluster)  [unwired: 2 out]
      }
      frame "Handle Error" {
      }
    }
    n155 = call <vilib>:"Simple Error Handler.vi"("error in (no error)"=w18) -> ()  [unwired: 4 in, 5 out]
  }
